vi "Thermometer.vi"(1 "Boolean":bool) -> (0 "Thermometer":dbl(slide) scale=0.0..100.0)   [LabVIEW 2015]
doc: "This VI measures temperature using the temperaturesensor on the DAQ Signal Accessory"
panel:
  # "Temp Scale"
  # "deg C"
  # "deg F"
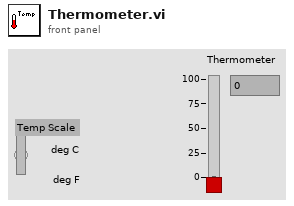
[diagram p1: front panel]
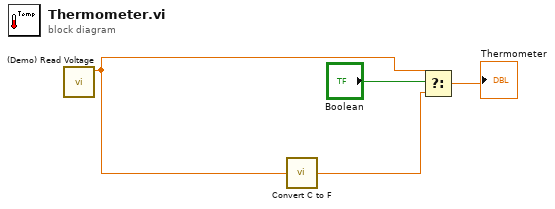
[diagram p0: block diagram]
diagram:
  n1 = call "(Demo) Read Voltage.vi"() -> ("voltage"=w2:dbl)  [unwired: 6 in, 1 out]
  n2 = call "Convert C to F.vi"("deg C"=w2) -> ("deg F"=w3:dbl)
  n3 = Select(t=w2, s="Boolean", f=w3) -> (s? t:f=→"Thermometer":dbl)
